vi "SetupDigitizer.vi"(0 "RIO Resource`":T3="PXI1Slot3", 1 "Trigger Level (V)":dbl, 2 "Delay after Trig (us)":dbl, 5 "Record Size":u16=1024, 7 "TIS Mode":T2=3 items=["TIS Mode (CH0 Only)"=1, "TIS Mode (CH1 Only)"=2, "Dual TIS Mode (CH0 and CH1)"=3], 9 "Clock Source":T1(ring)=enum."Internal Clock PLL On (IoModSyncClk)", 11 "error in":errorcluster, 12 "Trigger Type":enum8{"Software", "Data Edge"}(ring)) -> (4 "Default Configured?":bool, 6 "TIS Configured?":bool, 8 "Clocking Option Configured?":bool, 10 "Number of Elements":u16, 13 "range (Vpp)":dbl=1.3, 15 "error out":errorcluster)   [LabVIEW 2018]
uses:
  <vilib>/userdefined/High Color/nirio_resource_hc.ctl
  FPGA/Digitizer 5772/Controls/TIS Mode.ctl
  <vilib>/Utility/error.llb/Error Cluster From Error Code.vi
  <vilib>/rvi/errors/niLvFpgaAdjustHostInterfaceError.vi
  <vilib>/FPGAPlugInAG/Dynamic/niLvFpga_Close_Dynamic.vi
  <vilib>/rvi/interface/nirviReadWriteControl/nirviReadWriteControl.xnode
  <vilib>/rvi/interface/nirviCloseFPGA/nirviCloseFPGA.xnode
  NiFpgaLv.dll
  <vilib>/rvi/interface/Simulation/niFpgaSimulationCallBeginRW.vi
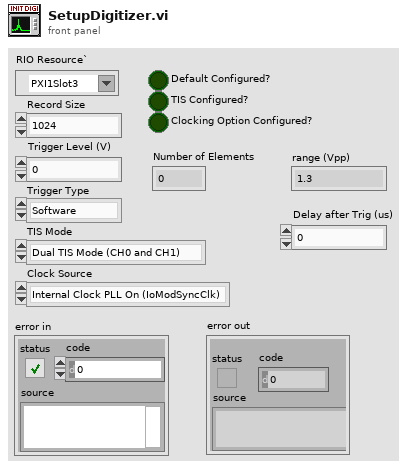
[diagram p1: front panel]
types:
  T1 = enum8{"Internal Clock PLL Off", "Internal Clock PLL On (REF IN)", "External Clock (CLK_IN)", "Internal Clock PLL On (IoModSyncClk)"}
  T2 = typedef "TIS Mode.ctl" = u16
  T3 = typedef "nirio_resource_hc.ctl" = tag
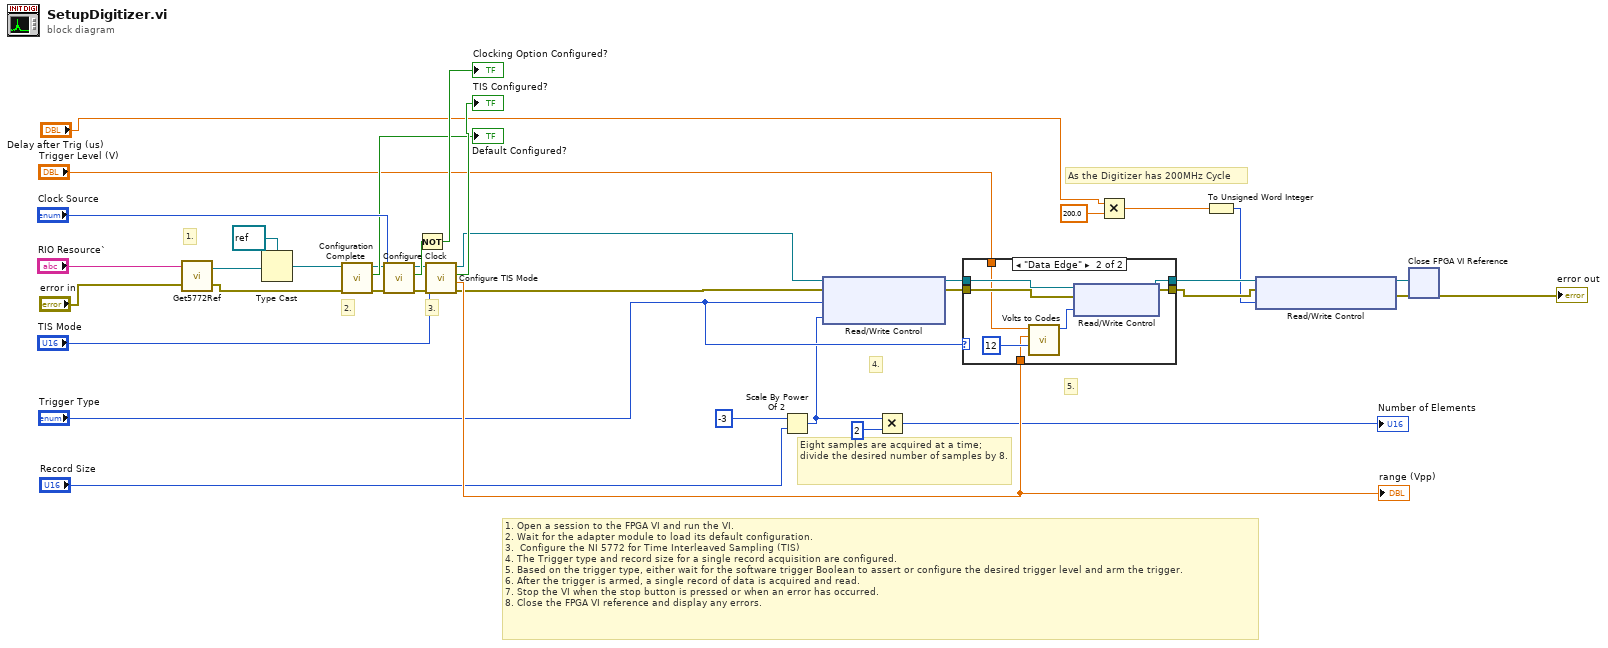
[diagram p0: block diagram]
diagram:
  # "As the Digitizer has 200MHz Cycle"
  # "Eight samples are acquired at a time; divide the desired number of samples by 8."
  # "5."
  # "4."
  # "3."
  # "2."
  # "1."
  # "1. Open a session to the FPGA VI and run the VI.\n2. Wait for the adapter module to load its default configuration.\n3.  Configure the NI 5772 for Time Interleaved Sampling (TIS)\n4. The Trigger type and record size for a single record acquisition are configured.\n5. Based on the trigger type, either wait for the software trigger Boolean to assert or configure the desired trigger level and arm the trigger.\n6. After the trigger is armed, a single record of data is acquired and read.\n7. Stop the VI when the stop button is pressed or when an error has occurred.  \n8. Close the FPGA VI reference and display any errors."
  n1 = call "Get5772Ref.vi"("error in (no error)"="error in", "RIO Device IN"="RIO Resource`") -> ("error out"=w1:errorcluster, "FPGA VI Reference Out"=w4:refnum<k20>)
  n2 = Type Cast(type=refnum<k20> refnum ("FPGA VI Reference Out"), x=w4) -> (*(type *) &x=w13:refnum<k20>)
  n3 = call "Configuration Complete.vi"("error in"=w1, "FPGA VI Reference In"=w13) -> ("error out"=w24:errorcluster, "Configured?"=→"Default Configured?":bool, "FPGA VI Reference Out"=w25:refnum<k20>)  [unwired: 7 out]
  n4 = call "Configure Clock.vi"("error in"=w24, "Clock Source"="Clock Source", "FPGA VI Reference In"=w25) -> ("error out"=w26:errorcluster, "Configuration Error"=w32:bool, "FPGA VI Reference Out"=w30:refnum<k20>)  [unwired: 6 in]
  n5 = Not(x=w32) -> (.not. x?=→"Clocking Option Configured?":bool)
  n6 = call "Configure TIS Mode.vi"("error in"=w26, "TIS Mode"="TIS Mode", "FPGA VI Reference In"=w30) -> ("error out"=w27:errorcluster, "range (Vpp)"=w34:dbl, "TIS Configured?"=→"TIS Configured?":bool, "FPGA VI Reference Out"=w28:refnum<k20>)  [unwired: 5 in]
  "range (Vpp)" <- w34
  n7 = Scale By Power Of 2(n=-3, x="Record Size") -> (x*2^n=w18:u16)
  n8 = xnode "Read/Write Control"("FPGA VI Reference In"=w28, "error in"=w27, "Trigger Type"="Trigger Type", "Samples Per Trigger"=w18) -> ("FPGA VI Reference Out"=w21:refnum<k20>, "error out"=w20:errorcluster)
  n9 = Multiply(x=w18, y=u16 2) -> (x*y=→"Number of Elements":u16)
  n10 = case shown="\"Data Edge\"" "Trigger Type" {
    tunnel: w21 -> [w39 w47]
    tunnel: w20 -> [w38 w46]
    tunnel: [w39 w45] -> w14
    tunnel: [w38 w44] -> w7
    tunnel: w34 -> [_ w41]
    tunnel: "Trigger Level (V)" -> [_ w40]
    frame "Software", Default {
    }
    frame "Data Edge" {
      n11 = call "Volts to Codes.vi"("Number of Bits"=i16 12, "range (Vpp)"=w41, "Data In"=w40) -> ("Data Out"=w42:i16)  [unwired: 8 out]
      n12 = xnode "Read/Write Control"("FPGA VI Reference In"=w47, "error in"=w46, "Trigger Level"=w42) -> ("FPGA VI Reference Out"=w45:refnum<k20>, "error out"=w44:errorcluster)
    }
  }
  n13 = Multiply(x="Delay after Trig (us)", y=200.0) -> (x*y=w10:dbl)
  n14 = To Unsigned Word Integer(number=w10) -> (unsigned 16bit integer=w5:u16)
  n15 = xnode "Read/Write Control"("FPGA VI Reference In"=w14, "error in"=w7, "Delay after Trig [cycles]"=w5) -> ("FPGA VI Reference Out"=w8:refnum<k20>, "error out"=w6:errorcluster)
  n16 = xnode "Close FPGA VI Reference"("FPGA VI Reference In"=w8, "error in"=w6) -> ("error out"=→"error out":errorcluster)
